vi "Demo_Write_Output.vi"(6 "OUTPUT STATUS":string(combo)="L", 7 "Mode":enum16{"Single", "All"}(ring), 8 "error in (no error)":errorcluster, 9 "Select Output":string(combo)="OP1", 10 "CID IN":string, 11 "Output Status":string[](array[string])) -> (0 "error out":errorcluster, 2 "JSON STRING OUT":string, 3 "Topic":string)   [LabVIEW 2017]
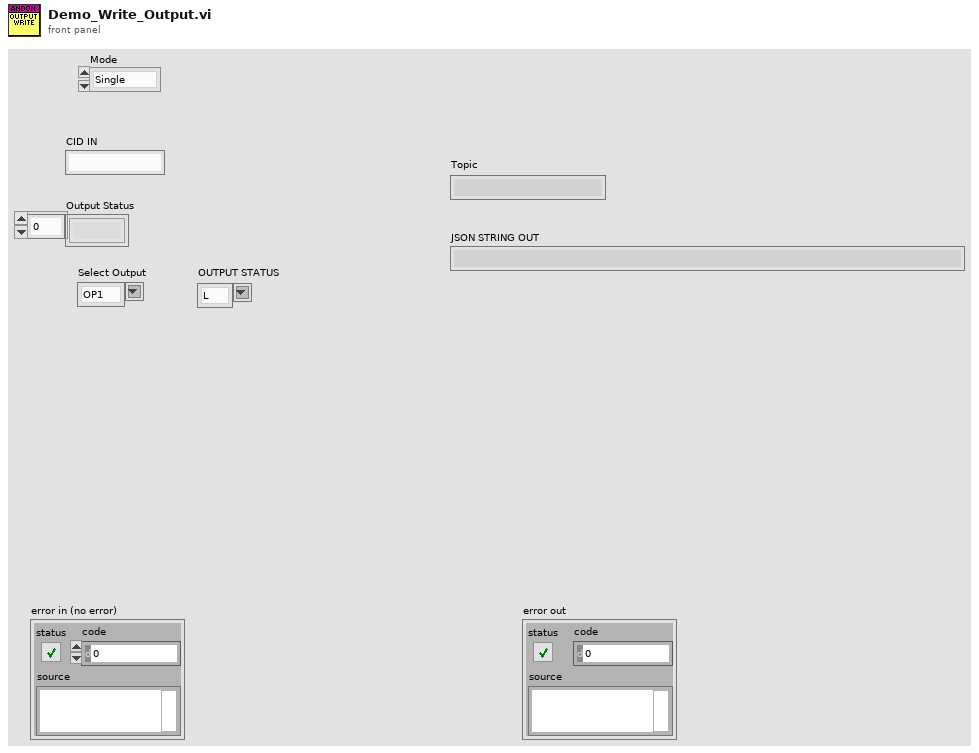
[diagram p1: front panel]
types:
  T1 = cluster{"MID":string, "MODE":string, "OP1":string, "OP2":string, "OP3":string, "OP4":string, "OP5":string, "OP6":string, "OP7":string, "OP8":string}
  T2 = cluster{"MID":string, "MODE":string, "OP1":string}
  T3 = cluster{"MID":string, "MODE":string, "OP2":string}
  T4 = cluster{"MID":string, "MODE":string, "OP3":string}
  T5 = cluster{"MID":string, "MODE":string, "OP4":string}
  T6 = cluster{"MID":string, "MODE":string, "OP5":string}
  T7 = cluster{"MID":string, "MODE":string, "OP6":string}
  T8 = cluster{"MID":string, "MODE":string, "OP7":string}
  T9 = cluster{"MID":string, "MODE":string, "OP8":string}
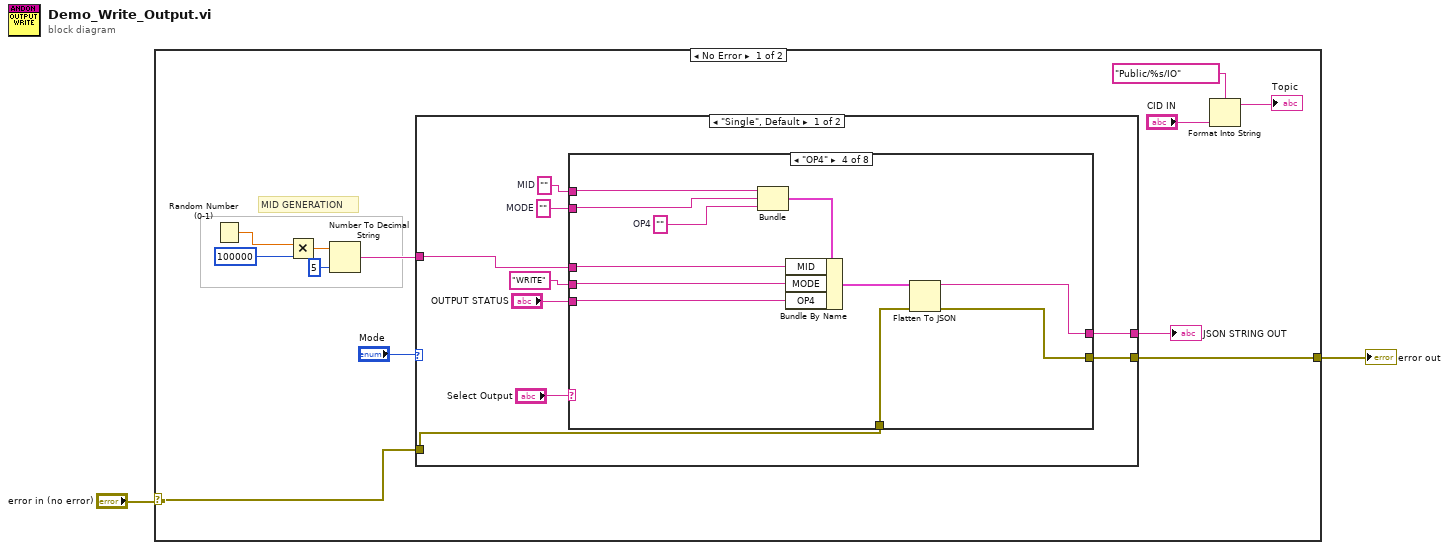
[diagram p0: block diagram]
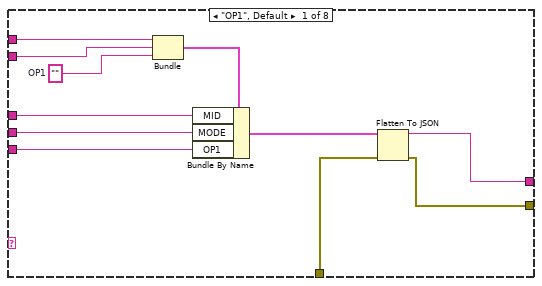
[diagram p2: hidden frame]
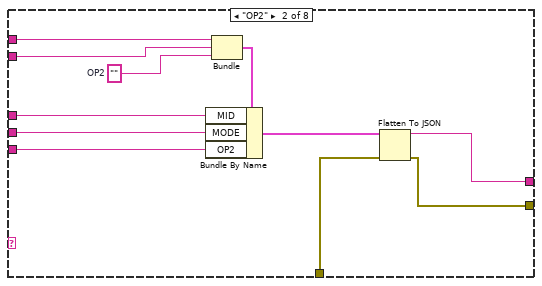
[diagram p3: hidden frame]
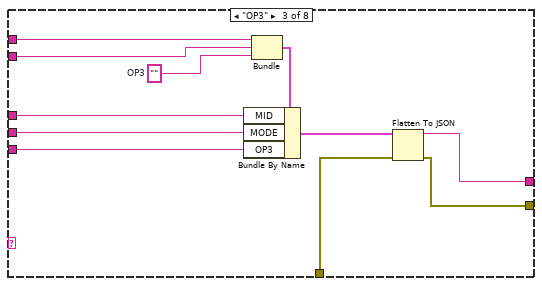
[diagram p4: hidden frame]
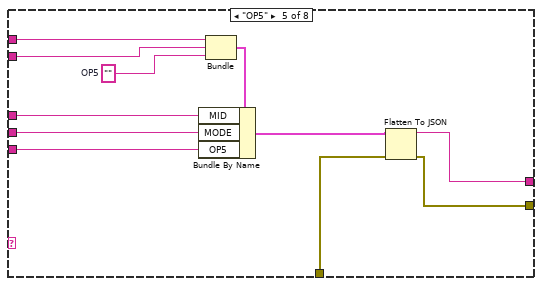
[diagram p5: hidden frame]
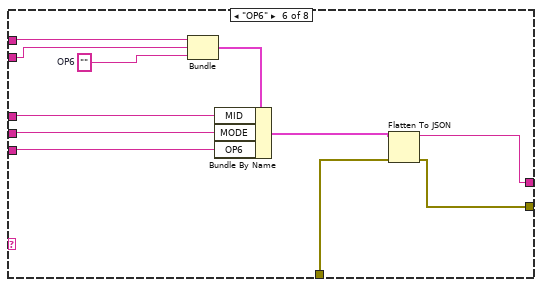
[diagram p6: hidden frame]
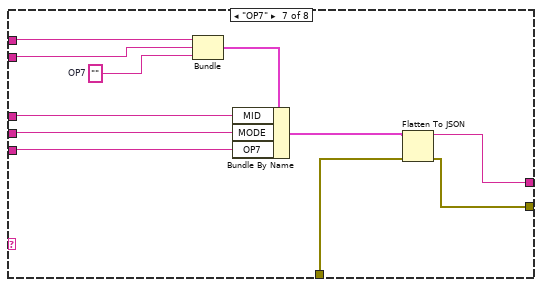
[diagram p7: hidden frame]
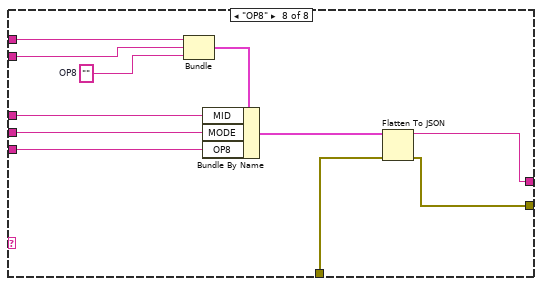
[diagram p8: hidden frame]
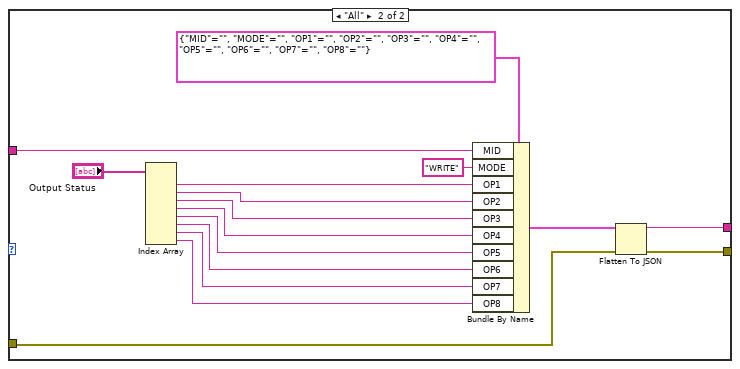
[diagram p9: hidden frame]
diagram:
  n1 = case shown="No Error" "error in (no error)" {
    selector: "error in (no error)" -> [w7 w128]
    tunnel: [w6 w128] -> w2
    frame No Error {
      # "MID GENERATION"
      n2 = Random Number (0-1)() -> (number: 0 to 1=w13:dbl)
      n3 = Multiply(x=w13, y=100000) -> (x*y=w12:dbl)
      n4 = Number To Decimal String(number=w12, width (-)=i16 5) -> (decimal integer string=w9:string)
      n5 = case shown="\"Single\", Default" "Mode" {
        tunnel: w9 -> [w20 w125]
        tunnel: [w17 w123] -> w8
        tunnel: w7 -> [w16 w122]
        tunnel: [w15 w121] -> w6
        frame "Single", Default {
          w21 = ""  # MODE
          w22 = ""  # MID
          n6 = case shown="\"OP4\"" "Select Output" {
            tunnel: w22 -> [w34 w43 w51 w62 w76 w87 w98 w109]
            tunnel: w21 -> [w33 w42 w50 w61 w75 w86 w97 w108]
            tunnel: w20 -> [w30 w41 w54 w65 w74 w85 w96 w107]
            tunnel: "OUTPUT STATUS" -> [w29 w39 w52 w63 w72 w83 w94 w105]
            tunnel: "WRITE" ("MODE") -> [w28 w40 w53 w64 w73 w84 w95 w106]
            tunnel: [w24 w35 w46 w59 w68 w79 w90 w101] -> w17
            tunnel: w16 -> [w26 w37 w48 w58 w70 w81 w92 w103]
            tunnel: [w25 w36 w47 w57 w69 w80 w91 w102] -> w15
            frame "OP1", Default {
              w32 = ""  # OP1
              n7 = Bundle("MID"=w34, "MODE"=w33, "OP1"=w32) -> (w31:T2)  [unwired: 1 in]
              n8 = Bundle By Name(cluster=w31, "MID"=w30, "MODE"=w28, "OP1"=w29) -> (w27:T2)
              n9 = Flatten To JSON(anything=w27, error in (no error)=w26) -> (JSON string=w24:string, 11:w25:errorcluster)  [unwired: 1 in]
            }
            frame "OP2" {
              w45 = ""  # OP2
              n10 = Bundle("MID"=w43, "MODE"=w42, "OP2"=w45) -> (w44:T3)  [unwired: 1 in]
              n11 = Bundle By Name(cluster=w44, "MID"=w41, "MODE"=w40, "OP2"=w39) -> (w38:T3)
              n12 = Flatten To JSON(anything=w38, error in (no error)=w37) -> (JSON string=w35:string, 11:w36:errorcluster)  [unwired: 1 in]
            }
            frame "OP3" {
              w56 = ""  # OP3
              n13 = Bundle("MID"=w51, "MODE"=w50, "OP3"=w56) -> (w55:T4)  [unwired: 1 in]
              n14 = Bundle By Name(cluster=w55, "MID"=w54, "MODE"=w53, "OP3"=w52) -> (w49:T4)
              n15 = Flatten To JSON(anything=w49, error in (no error)=w48) -> (JSON string=w46:string, 11:w47:errorcluster)  [unwired: 1 in]
            }
            frame "OP4" {
              w67 = ""  # OP4
              n16 = Bundle("MID"=w62, "MODE"=w61, "OP4"=w67) -> (w66:T5)  [unwired: 1 in]
              n17 = Bundle By Name(cluster=w66, "MID"=w65, "MODE"=w64, "OP4"=w63) -> (w60:T5)
              n18 = Flatten To JSON(anything=w60, error in (no error)=w58) -> (JSON string=w59:string, 11:w57:errorcluster)  [unwired: 1 in]
            }
            frame "OP5" {
              w78 = ""  # OP5
              n19 = Bundle("MID"=w76, "MODE"=w75, "OP5"=w78) -> (w77:T6)  [unwired: 1 in]
              n20 = Bundle By Name(cluster=w77, "MID"=w74, "MODE"=w73, "OP5"=w72) -> (w71:T6)
              n21 = Flatten To JSON(anything=w71, error in (no error)=w70) -> (JSON string=w68:string, 11:w69:errorcluster)  [unwired: 1 in]
            }
            frame "OP6" {
              w89 = ""  # OP6
              n22 = Bundle("MID"=w87, "MODE"=w86, "OP6"=w89) -> (w88:T7)  [unwired: 1 in]
              n23 = Bundle By Name(cluster=w88, "MID"=w85, "MODE"=w84, "OP6"=w83) -> (w82:T7)
              n24 = Flatten To JSON(anything=w82, error in (no error)=w81) -> (JSON string=w79:string, 11:w80:errorcluster)  [unwired: 1 in]
            }
            frame "OP7" {
              w100 = ""  # OP7
              n25 = Bundle("MID"=w98, "MODE"=w97, "OP7"=w100) -> (w99:T8)  [unwired: 1 in]
              n26 = Bundle By Name(cluster=w99, "MID"=w96, "MODE"=w95, "OP7"=w94) -> (w93:T8)
              n27 = Flatten To JSON(anything=w93, error in (no error)=w92) -> (JSON string=w90:string, 11:w91:errorcluster)  [unwired: 1 in]
            }
            frame "OP8" {
              w111 = ""  # OP8
              n28 = Bundle("MID"=w109, "MODE"=w108, "OP8"=w111) -> (w110:T9)  [unwired: 1 in]
              n29 = Bundle By Name(cluster=w110, "MID"=w107, "MODE"=w106, "OP8"=w105) -> (w104:T9)
              n30 = Flatten To JSON(anything=w104, error in (no error)=w103) -> (JSON string=w101:string, 11:w102:errorcluster)  [unwired: 1 in]
            }
          }
        }
        frame "All" {
          n31 = Index Array(array="Output Status") -> (element #1=w120:string, element #2=w118:string, element #3=w112:string, element #4=w117:string, element #5=w116:string, element #6=w115:string, element #7=w114:string, element #8=w113:string)  [unwired: 8 in]
          n32 = Bundle By Name(cluster=T1 {"MID"="", "MODE"="", "OP1"="", "OP2"="", "OP3"="", "OP4"="", "OP5"="", "OP6"="", "OP7"="", "OP8"=""}, "MID"=w125, "MODE"="WRITE", "OP1"=w120, "OP2"=w118, "OP3"=w112, "OP4"=w117, "OP5"=w116, "OP6"=w115, "OP7"=w114, "OP8"=w113) -> (w124:T1)
          n33 = Flatten To JSON(anything=w124, error in (no error)=w122) -> (JSON string=w123:string, 11:w121:errorcluster)  [unwired: 1 in]
        }
      }
      "JSON STRING OUT" <- w8
      n34 = Format Into String(format string="Public/%s/IO" ("Topic"), "CID IN") -> (resulting string=→"Topic":string)  [unwired: 2 in, 1 out]
    }
    frame Error {
    }
  }
  "error out" <- w2
